vi "Index_tv_ts_td.vi"(3 "计算参数 in":T1, 5 "Array in":dbl[](array[numeric])) -> (0 "计算参数 out":T1, 2 "Array out":dbl[](array[numeric]))   [LabVIEW 2013]
doc: "此程序以行程数组和计算参数的簇作为输入，计算tv ts td的索引值。"
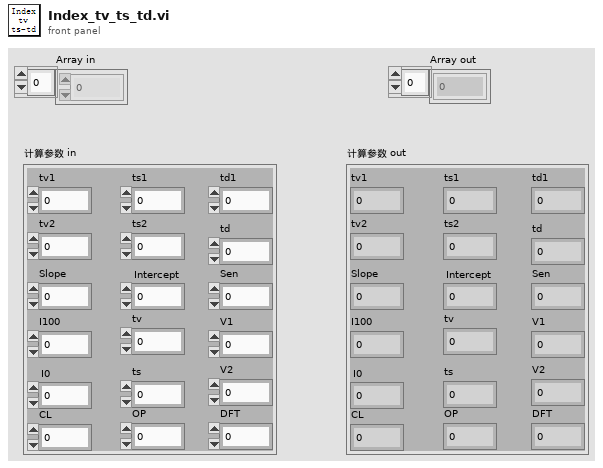
[diagram p1: front panel]
types:
  T1 = cluster{"tv1":dbl, "tv2":dbl, "tv":dbl, "ts1":dbl, "ts2":dbl, "ts":dbl, "td1":dbl, "td":dbl, "Slope":dbl, "Intercept":dbl, "I100":dbl, "I0":dbl, "Sen":dbl, "V1":dbl, "V2":dbl, "CL":dbl, "OP":dbl, "DFT":dbl}
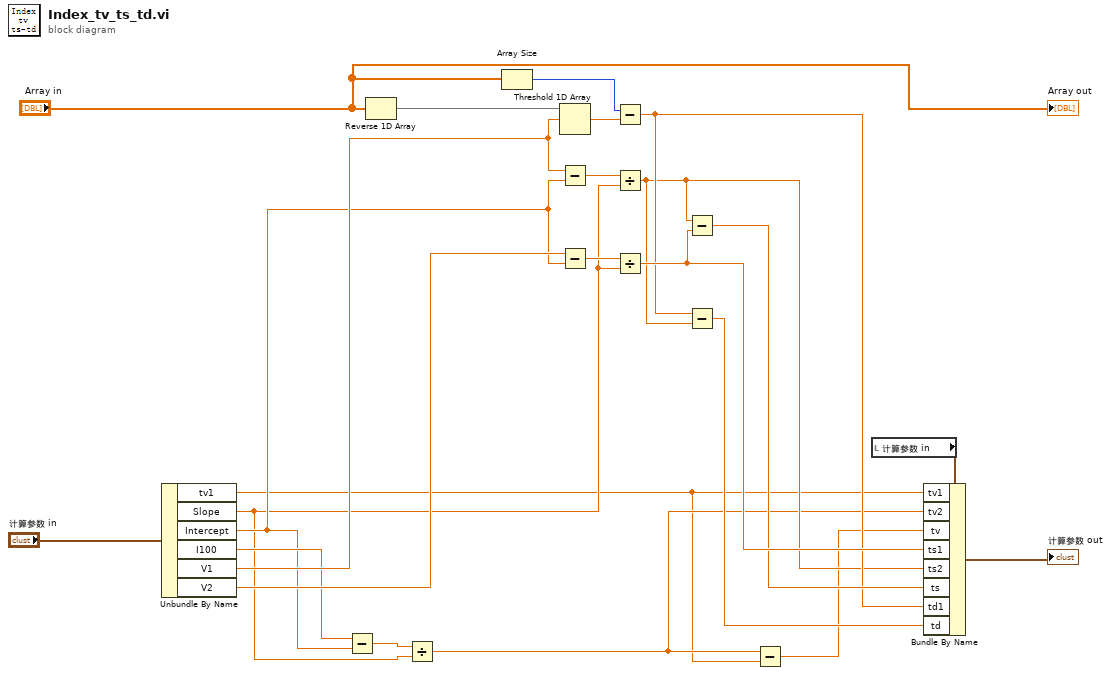
[diagram p0: block diagram]
diagram:
  n1 = Unbundle By Name("计算参数 in") -> ("tv1"=w2:dbl, "Slope"=w4:dbl, "Intercept"=w6:dbl, "I100"=w7:dbl, "V1"=w15:dbl, "V2"=w14:dbl)
  n2 = Subtract(x=w7, y=w6) -> (x-y=w5:dbl)
  n3 = Reverse 1D Array(array="Array in") -> (reversed array=w22:dbl[])
  n4 = Divide(x=w5, y=w4) -> (x/y=w3:dbl)
  n5 = Array Size(array="Array in") -> (size(s)=w16:i32)
  n6 = Threshold 1D Array(2:w15, 3:w22) -> (0:w23:dbl)  [unwired: 1 in]
  n7 = Subtract(x=w15, y=w6) -> (x-y=w20:dbl)
  n8 = Subtract(x=w14, y=w6) -> (x-y=w21:dbl)
  n9 = Subtract(x=w16, y=w23) -> (x-y=w9:dbl)
  n10 = Divide(x=w20, y=w4) -> (x/y=w8:dbl)
  n11 = Divide(x=w21, y=w4) -> (x/y=w12:dbl)
  n12 = Subtract(x=w8, y=w12) -> (x-y=w11:dbl)
  n13 = Subtract(x=w9, y=w8) -> (x-y=w10:dbl)
  n14 = Subtract(x=w3, y=w2) -> (x-y=w1:dbl)
  n15 = local read "计算参数 in"() -> (w17:T1)
  n16 = Bundle By Name(cluster=w17, "tv1"=w2, "tv2"=w3, "tv"=w1, "ts1"=w12, "ts2"=w8, "ts"=w11, "td1"=w9, "td"=w10) -> (→"计算参数 out":T1)
  "Array out" <- "Array in"
